vi "close.vi"(8 "error in":errorcluster, 11 "module in":refnum<class "TBM module execution interface.lvclass">) -> (0 "error out":errorcluster)   [LabVIEW 2013, in "TBM module execution interface.lvclass"]
doc: "Provides an interface for terminating a module instance. While this interface performs no operations, a child should close and deallocate any open references or memory."
uses:
  TBM module execution interface.lvclass
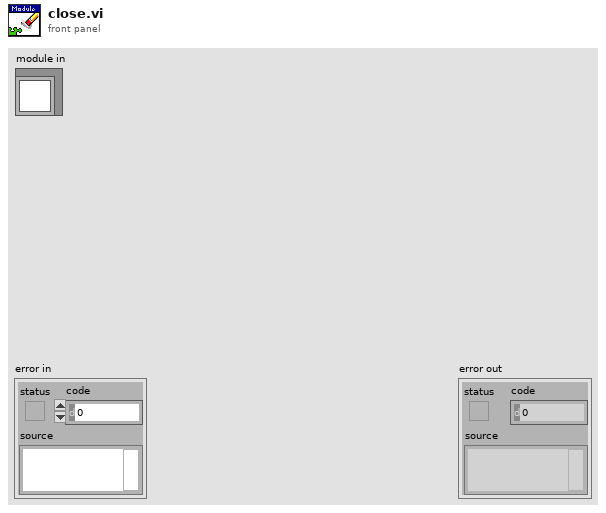
[diagram p1: front panel]
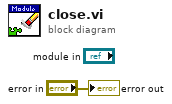
[diagram p0: block diagram]
diagram:
  "error out" <- "error in"
